vi "Write Serial Data in tdms.vi"(7 "Command":T1, 8 "error in (no error)":errorcluster, 11 "Data":string) -> (0 "error out":errorcluster)   [LabVIEW 2016, in "Serial Hardware.lvlib"]
uses:
  Serial Hardware.lvlib
  Write Data Command.ctl
  User Interface/Create Path Command.ctl
  User Interface/User Interface.lvlib
panel:
  in  "Channel name":string[](array[string])
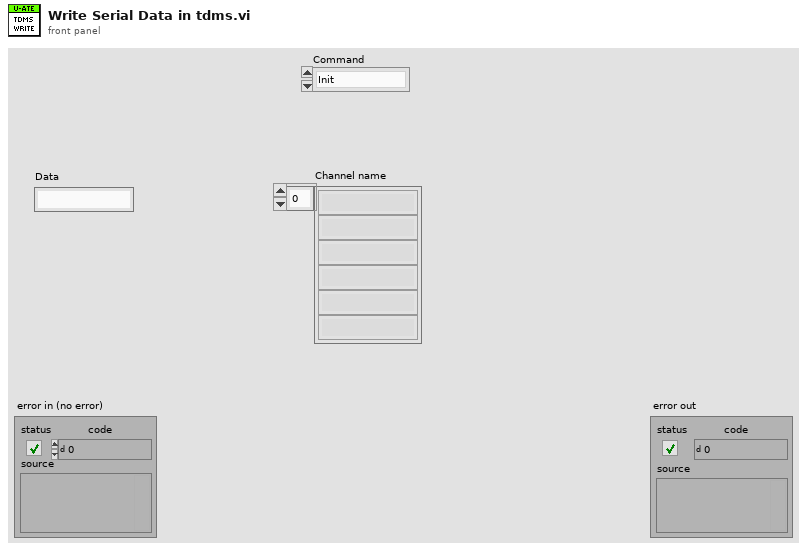
[diagram p1: front panel]
types:
  T1 = typedef "Serial Hardware.lvlib/Write Data Command.ctl" = enum16{"Init", "Read", "Write", "close"}
  T2 = typedef "User Interface.lvlib/Create Path Command.ctl" = enum16{"Authentication", "Hardware", "Configuration", "Calibration", "Instrument", "Test Description", "Serial Data", "ARINC Data", "CAN Data", "Data", "Report", "Action log", "Error Log"}
  T3 = enum16{"open", "open or create", "create or replace", "create", "open (read-only)"}
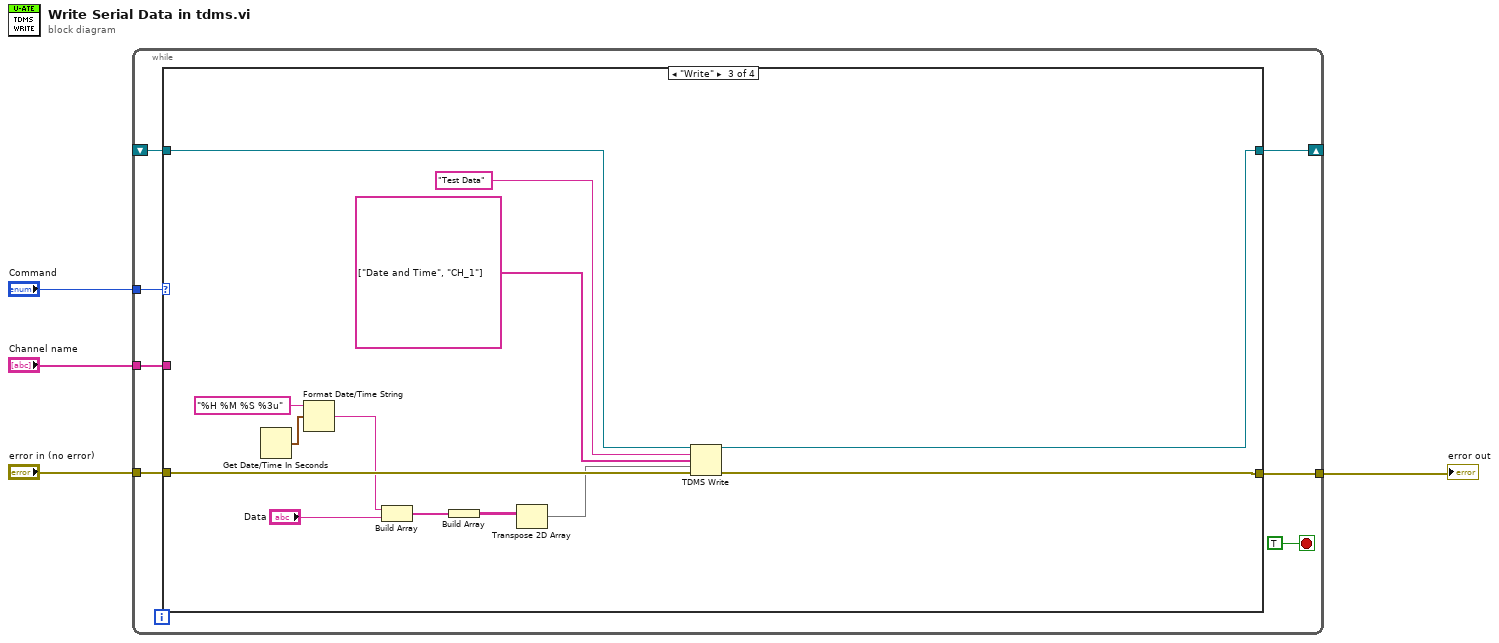
[diagram p0: block diagram]
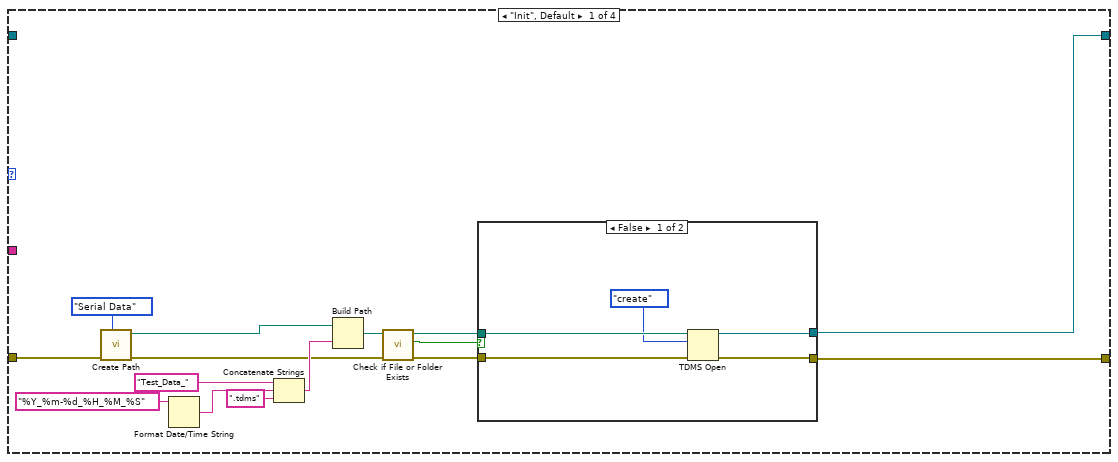
[diagram p2: hidden frame]
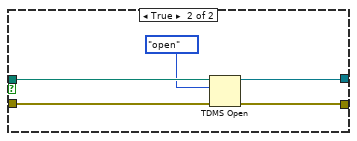
[diagram p3: hidden frame]
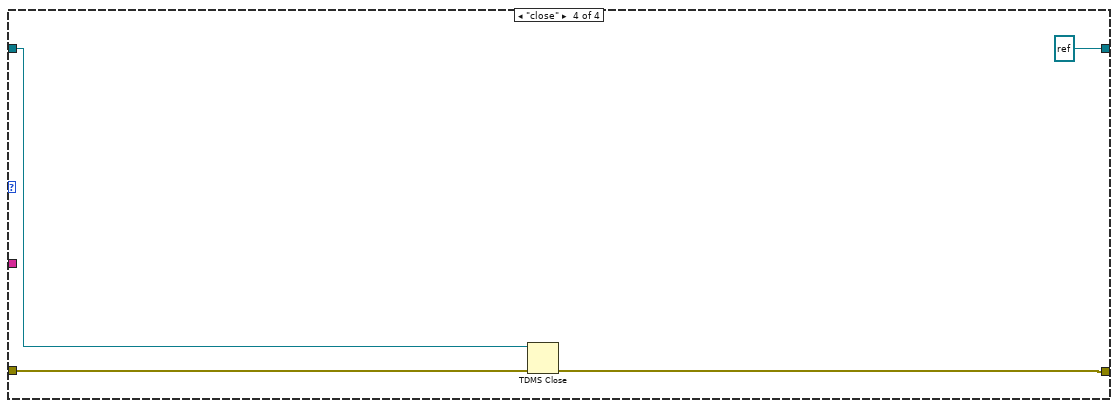
[diagram p5: hidden frame]
diagram:
  n1 = while {
    tunnel: "error in (no error)" -> [w10]
    tunnel: [w9] -> w3
    shift-right: [w8] -> _
    shift-left: _ -> [w7]
    tunnel: "Channel name" -> [w6]
    tunnel: "Command" -> [w5]
    stop <- TRUE stop-if-true
    n2 = case shown="\"Write\"" w5 {
      tunnel: w10 -> [w26 w37 w51 w55]
      tunnel: [w13 w37 w48 w54] -> w9
      tunnel: [w12 w38 w49 refnum<k34> refnum ("tdms file out")] -> w8
      tunnel: w7 -> [_ w38 w50 w53]
      tunnel: w6 -> [_ _ _ _]
      frame "Init", Default {
        n3 = call "Create Path.vi"("Path Command"=Create_Path_Command."Serial Data", "error in (no error)"=w26) -> ("error out"=w14:errorcluster, "created path"=w20:path)  [unwired: 8 in]
        n4 = Format Date/Time String(time format string (%c)="%Y_%m-%d_%H_%M_%S") -> (date/time string=w18:string)  [unwired: 2 in]
        n5 = Concatenate Strings("Test_Data_" ("string"), w18, ".tdms" ("string")) -> (w16:string)
        n6 = Build Path(base path=w20, name or relative path=w16) -> (appended path=w15:path)
        n7 = call <vilib>:"Check if File or Folder Exists.vi"("error in (no error)"=w14, "path"=w15) -> ("error out"=w24:errorcluster, "file or folder exists?"=w23:bool, "dup path"=w22:path)  [unwired: 7 in]
        n8 = case shown="False" w23 {
          tunnel: w24 -> [w30 w36]
          tunnel: w22 -> [w31 w35]
          tunnel: [w28 w33] -> w13
          tunnel: [w27 w34] -> w12
          frame False {
            n9 = TDMS Open(8:w30, 10:T3."create" ("operation (0:open)"), 11:w31) -> (0:w28:errorcluster, 3:w27:refnum<k34>)  [unwired: 4 in]
          }
          frame True {
            n10 = TDMS Open(8:w36, 10:T3."open" ("operation (0:open)"), 11:w35) -> (0:w33:errorcluster, 3:w34:refnum<k34>)  [unwired: 4 in]
          }
        }
      }
      frame "Read" {
      }
      frame "Write" {
        n11 = Get Date/Time In Seconds() -> (seconds since 1Jan1904=w44:timestamp)
        n12 = Format Date/Time String(time format string (%c)="%H %M %S %3u", seconds (now)=w44) -> (date/time string=w42:string)  [unwired: 1 in]
        n13 = Build Array(w42, "Data") -> (w41:string[])
        n14 = Build Array(w41) -> (w39:string[][])
        n15 = Transpose 2D Array(2D array=w39) -> (transposed array=w40:string[][])
        n16 = TDMS Write(0:w50, 5:"Test Data", 7:string[] ["Date and Time", "CH_1"], 9:w40, 11:w51) -> (4:w49:refnum<k34>, 15:w48:errorcluster)  [unwired: 1 in, 2 out]
      }
      frame "close" {
        n17 = TDMS Close(8:w55, 11:w53) -> (0:w54:errorcluster)  [unwired: 1 out]
      }
    }
  }
  "error out" <- w3
